vi "Array_Pair_Multiplier.vi"() -> ()   [LabVIEW 2020]
panel:
  out "MULTIPLIED ARRAY":dbl[](array[numeric])
  in  "Input Array":dbl[](array[numeric])
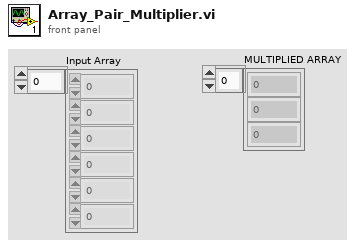
[diagram p1: front panel]
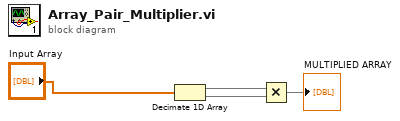
[diagram p0: block diagram]
diagram:
  n1 = Decimate 1D Array("Input Array") -> (w3:dbl[], w2:dbl[])
  n2 = Multiply(x=w3, y=w2) -> (x*y=→"MULTIPLIED ARRAY":dbl[])
